vi "Acquire.vi"(8 "error in (no error)":errorcluster, 9 "Initialize":bool, 10 "Reply to":refnum<class "Result Reply Msg.lvclass">, 11 "Measure Object in":refnum<class "da Base.lvclass">) -> (0 "error out":errorcluster, 3 "Measure Object out":refnum<class "da Base.lvclass">)   [LabVIEW 2016, in "da Base.lvclass"]
uses:
  da Base.lvclass
  Da Base Messages/Result Reply Msg/Result Reply Msg.lvclass
  da Base.lvclass/da Base.ctl
  Write Reply to.vi
  Write Active.vi
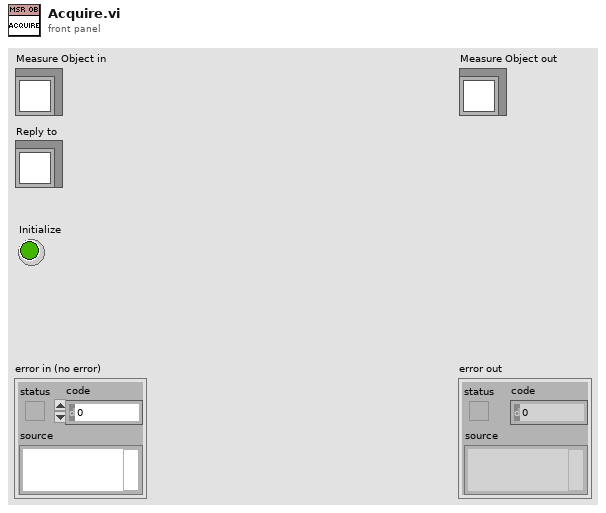
[diagram p1: front panel]
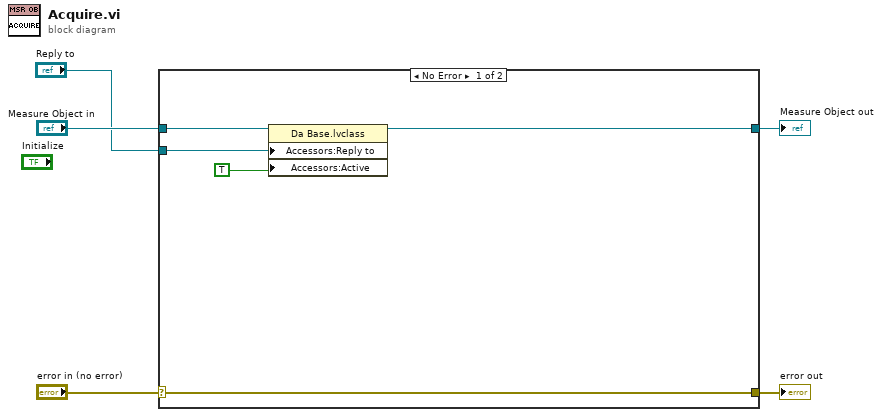
[diagram p0: block diagram]
diagram:
  n1 = case shown="No Error" "error in (no error)" {
    selector: "error in (no error)" -> [w9 w12]
    tunnel: [w9 w12] -> w4
    tunnel: [w8 w11] -> w2
    tunnel: "Measure Object in" -> [w10 w11]
    tunnel: "Reply to" -> [w7 _]
    frame No Error {
      n2 = property class="Da Base.lvclass"(reference=w10, "Accessors:Reply to"=w7, "Accessors:Active"=TRUE ("Active")) -> (reference out=w8:refnum<class "da Base.lvclass">)  [unwired: 1 in, 1 out]
    }
    frame Error {
    }
  }
  "error out" <- w4
  "Measure Object out" <- w2
